vi "Pre Launch Init.vi"(11 "Timed Loop Controller in":refnum<class "Reference Range Actor.lvclass">) -> (0 "error out":errorcluster, 3 "Timed Loop Controller out":refnum<class "Reference Range Actor.lvclass">)   [LabVIEW 2018, in "Reference Range.lvlib" / "Reference Range Actor.lvclass"]
uses:
  Reference Range Actor.lvclass
  Reference Range Actor.lvclass/Reference Range Actor.ctl
  Actor Monitor/Actor/Monitored Actor.lvclass
panel:
  in  "error in (no error)":errorcluster
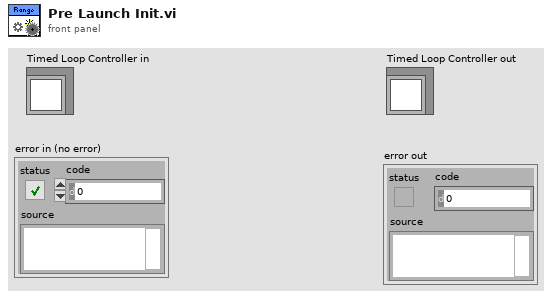
[diagram p1: front panel]
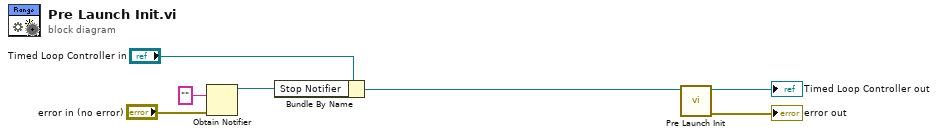
[diagram p0: block diagram]
diagram:
  n1 = Obtain Notifier(notification data type="", error in (no error)="error in (no error)") -> (notifier out=w3:refnum<notifier>)  [unwired: 2 in, 2 out]
  n2 = Bundle By Name(cluster="Timed Loop Controller in", "Stop Notifier"=w3) -> (w2:refnum<class "Reference Range Actor.lvclass">)
  n3 = call-parent "Pre Launch Init.vi"("Monitored Actor in"=w2) -> ("error out"=→"error out":errorcluster, "Monitored Actor out"=→"Timed Loop Controller out":refnum<class "Reference Range Actor.lvclass">)  [unwired: 9 in]
